vi "Insert_Rewire Terminal.vi"(8 "error in":errorcluster, 10 "New Terminal":refnum<vi>, 11 "Old Terminal":refnum<vi>) -> (0 "error out":errorcluster, 3 "Terminals Rewired?":bool)   [LabVIEW 2020]
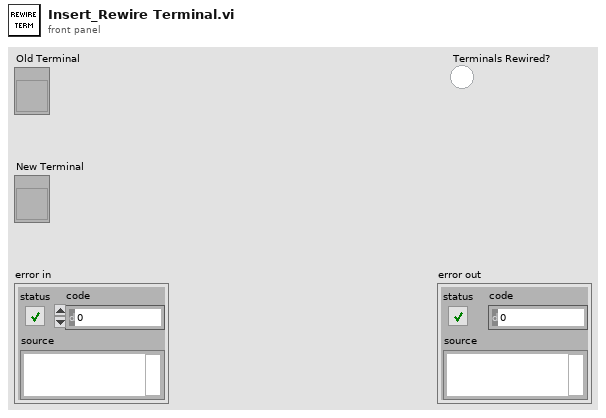
[diagram p1: front panel]
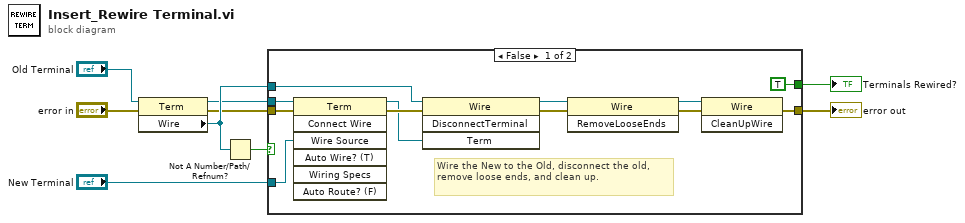
[diagram p0: block diagram]
diagram:
  n1 = property class="Term"(reference="Old Terminal", error in="error in") -> (reference out=w5:refnum<vi>, error out=w6:errorcluster, "Wire"=w7:refnum<vi>)
  n2 = Not A Number/Path/Refnum?(number/path/refnum=w7) -> (NaN/Path/Refnum?=w8:bool)
  n3 = case shown="False" w8 {
    tunnel: [w19 w22] -> w1
    tunnel: "New Terminal" -> [w18 _]
    tunnel: w5 -> [w17 _]
    tunnel: w6 -> [w16 w22]
    tunnel: w7 -> [w15 _]
    tunnel: [TRUE _] -> w9
    frame False {
      # "Wire the New to the Old, disconnect the old, remove loose ends, and clean up."
      n4 = invoke class="Term" method="Connect Wire"(reference=w17, error in=w16, "Wire Source"=w18) -> (reference out=w20:refnum<vi>, error out=w21:errorcluster)  [unwired: 4 in, 5 out]
      n5 = invoke class="Wire" method="DisconnectTerminal"(reference=w15, error in=w21, "Term"=w20) -> (reference out=w13:refnum<vi>, error out=w11:errorcluster)  [unwired: 1 in, 2 out]
      n6 = invoke class="Wire" method="RemoveLooseEnds"(reference=w13, error in=w11) -> (reference out=w12:refnum<vi>, error out=w10:errorcluster)  [unwired: 1 in, 1 out]
      n7 = invoke class="Wire" method="CleanUpWire"(reference=w12, error in=w10) -> (error out=w19:errorcluster)  [unwired: 1 in, 2 out]
    }
    frame True {
      # "The old input isn't wired, so no-op."
    }
  }
  "Terminals Rewired?" <- w9
  "error out" <- w1
